vi "DN4_GetErrorPosition.vi"(3 "error in (no error)":errorcluster, 4 "error code":i32, 5 "task in":i32=-1) -> (0 "error out":errorcluster)   [LabVIEW 2020]
uses:
  DAQNavi_LV.dll
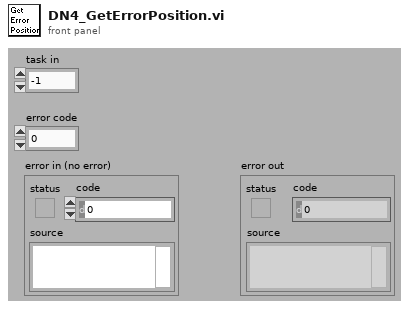
[diagram p1: front panel]
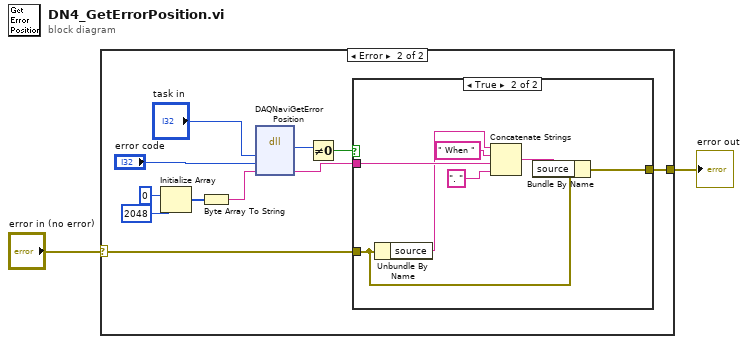
[diagram p0: block diagram]
diagram:
  n1 = case shown="Error" "error in (no error)" {
    selector: "error in (no error)" -> [w3 w9]
    tunnel: [w3 w5] -> w1
    frame No Error {
    }
    frame Error {
      n2 = Initialize Array(u8 0 ("element"), 2048 ("dimension size")) -> (w13:u8[])
      n3 = Byte Array To String(unsigned byte array=w13) -> (string=w14:string)
      n4 = dll-call lib="DAQNavi_LV.dll" fn="DAQNaviGetErrorPosition"("taskID"="task in", "err"="error code", "postion"=w14) -> ("return type"=w8:i8, "postion"=w6:string)  [unwired: 5 in, 2 out]
      n5 = Not Equal To 0?(x=w8) -> (x != 0?=w7:bool)
      n6 = case shown="True" w7 {
        tunnel: w9 -> [w15 w19]
        tunnel: w6 -> [_ w22]
        tunnel: [w15 w17] -> w5
        frame False {
        }
        frame True {
          n7 = Unbundle By Name(w19) -> ("source"=w16:string)
          n8 = Concatenate Strings(w16, " When " ("string"), w22, ". " ("string")) -> (w18:string)
          n9 = Bundle By Name(cluster=w19, "source"=w18) -> (w17:errorcluster)
        }
      }
    }
  }
  "error out" <- w1
